vi "Preview.vi"(8 "error in":errorcluster, 11 "VISA resource in":refnum<visa-resource-name>) -> (0 "error out":errorcluster, 3 "VISA resource out":refnum<visa-resource-name>)   [LabVIEW 2025]
panel:
  out "read buffer":string
  in  "Stop":bool
  out "Inductive sensor":i32(slide) scale=0.0..1023.0
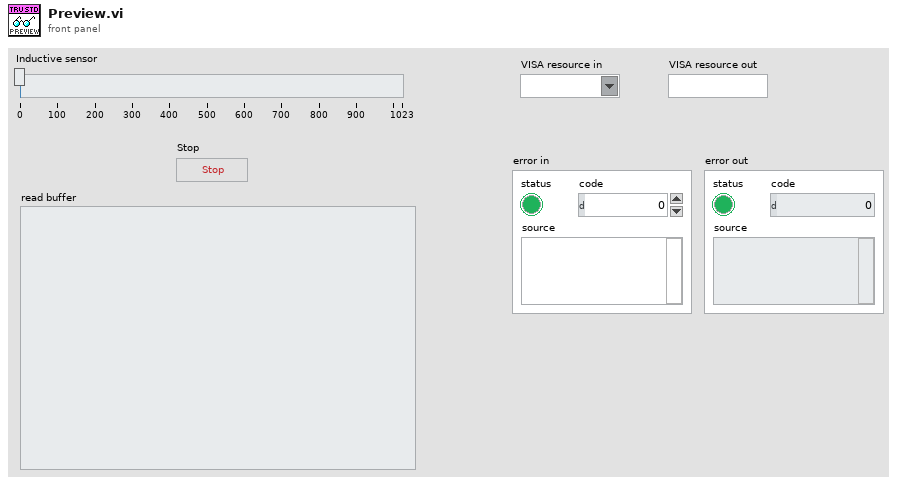
[diagram p1: front panel]
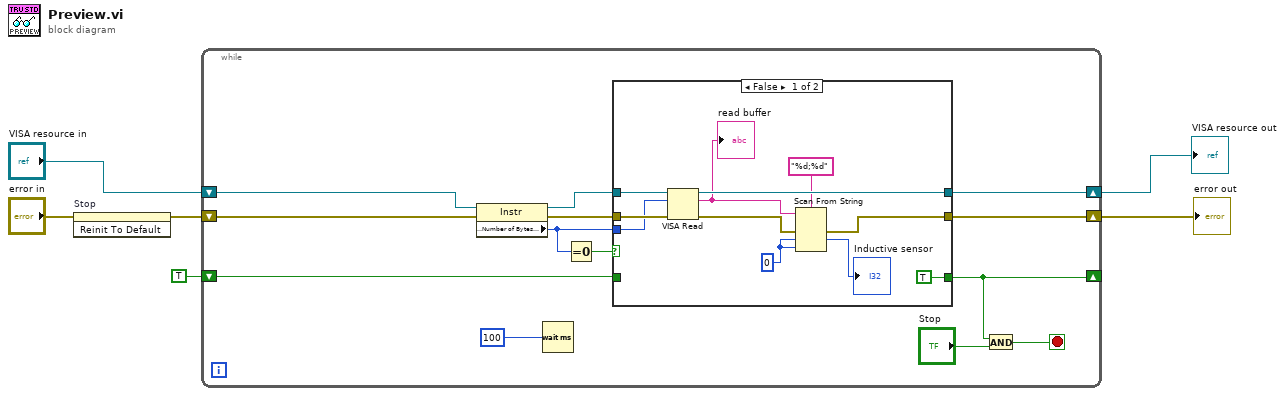
[diagram p0: block diagram]
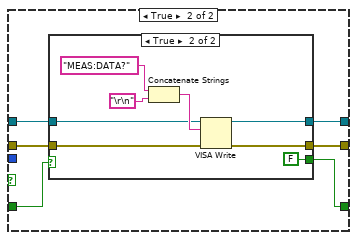
[diagram p2: hidden frame]
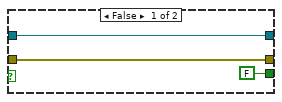
[diagram p3: hidden frame]
diagram:
  n1 = invoke on="Stop" class="Bool (strict)" method="Reinit To Default"(error in="error in") -> (error out=w1:errorcluster)  [unwired: 2 in, 2 out]
  n2 = while {
    shift-right: [w12] -> w5
    shift-left: "VISA resource in" -> [w13]
    shift-right: [w19] -> w4
    shift-left: w1 -> [w7]
    shift-right: [w10] -> _
    shift-left: TRUE -> [w11]
    stop <- w8 stop-if-true
    n3 = property class="Instr"(reference=w13, error in=w7) -> (reference out=w16:refnum<visa-resource-name>, error out=w17:errorcluster, "Serial Settings:Number of Bytes at Serial Port"=w15:u32)
    n4 = Wait (ms)(milliseconds to wait=u32 100) -> ()  [unwired: 1 out]
    n5 = Equal To 0?(x=w15) -> (x = 0?=w18:bool)
    n6 = case shown="False" w18 {
      tunnel: [w24 w34] -> w19
      tunnel: [w26 w33] -> w12
      tunnel: w17 -> [w30 w35]
      tunnel: w16 -> [w29 w36]
      tunnel: w15 -> [w28 _]
      tunnel: w11 -> [_ w32]
      tunnel: [TRUE w31] -> w10
      frame False {
        w21 = 0 ("default value 14")
        n7 = VISA Read(VISA resource name=w29, byte count=w28, error in (no error)=w30) -> (VISA resource name out=w26:refnum<visa-resource-name>, read buffer=w20:string, error out=w25:errorcluster)  [unwired: 1 out]
        "read buffer" <- w20
        n8 = Scan From String(format string="%d;%d", input string=w20, error in=w25, default 1=w21, default 2=w21) -> (error out=w24:errorcluster, output 1=→"Inductive sensor":i32)  [unwired: 2 in, 2 out]
      }
      frame True {
        n9 = case shown="True" w32 {
          tunnel: w36 -> [w38 w44]
          tunnel: w35 -> [w39 w43]
          tunnel: [w39 w42] -> w34
          tunnel: [w38 w41] -> w33
          tunnel: [FALSE FALSE] -> w31
          frame False {
          }
          frame True {
            n10 = Concatenate Strings("MEAS:DATA?" ("string"), "\r\n") -> (w45:string)
            n11 = VISA Write(VISA resource name=w44, write buffer=w45, error in (no error)=w43) -> (VISA resource name out=w41:refnum<visa-resource-name>, error out=w42:errorcluster)  [unwired: 1 out]
          }
        }
      }
    }
    n12 = And(x=w10, y="Stop") -> (x .and. y?=w8:bool)
  }
  "VISA resource out" <- w5
  "error out" <- w4
